vi "Polynomial Eigenvalues and Vectors (CDB).vi"(10 "output option":i32(ring)=1 items=["eigenvalues", "eigenvalues & vectors"], 11 "Input Matrices":cdb[][][](array[numeric])) -> (0 "error":i32, 2 "Eigenvectors":T1, 3 "Eigenvalues":cdb[](array[numeric]))   [LabVIEW 2010, in "NI_AALPro.lvlib"]
doc: "Solves the polynomial eigenvalue problem. Wire data to the <B>Input Matrices</B> input to determine the polymorphic instance to use or manually select the instance."
uses:
  NI_AALPro.lvlib
  ComplexMatrix.ctl
  NI_Matrix.lvlib
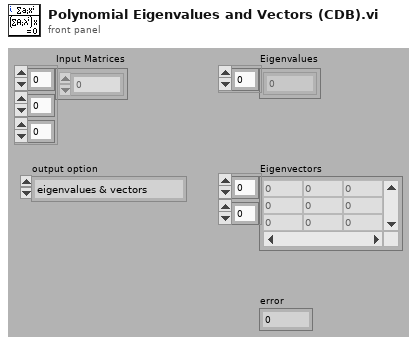
[diagram p1: front panel]
types:
  T1 = typedef "NI_Matrix.lvlib/ComplexMatrix.ctl" = cdb[][]
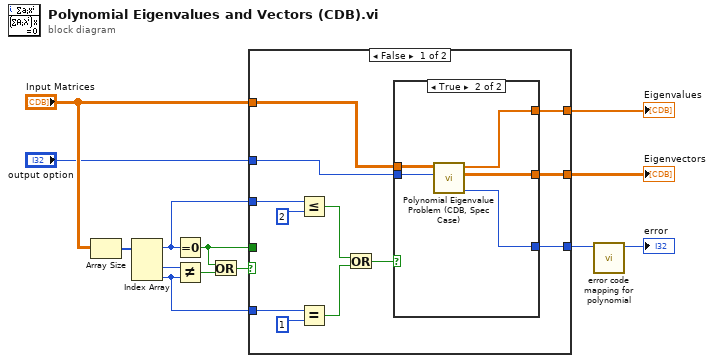
[diagram p0: block diagram]
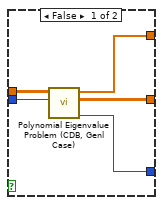
[diagram p2: hidden frame]
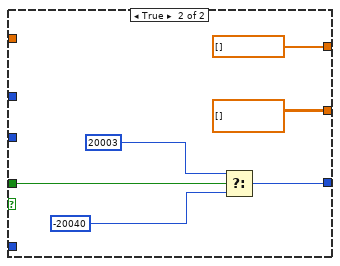
[diagram p3: hidden frame]
diagram:
  n1 = Array Size(array="Input Matrices") -> (size(s)=w13:i32[])
  n2 = Index Array(array=w13) -> (element #1=w7:i32, element #2=w12:i32, element #3=w8:i32)  [unwired: 3 in]
  n3 = Equal To 0?(x=w7) -> (x = 0?=w9:bool)
  n4 = Not Equal?(x=w12, y=w8) -> (x != y?=w11:bool)
  n5 = Or(x=w9, y=w11) -> (x .or. y?=w10:bool)
  n6 = case shown="False" w10 {
    tunnel: w9 -> [_ w41]
    tunnel: [w15 w38] -> w2
    tunnel: [w17 cdb[] [] ("Eigenvectors")] -> w4
    tunnel: [w16 cdb[][] [] ("Eigenvectors")] -> w5
    tunnel: "Input Matrices" -> [w23 _]
    tunnel: w8 -> [w25 _]
    tunnel: w7 -> [w22 _]
    tunnel: "output option" -> [w14 _]
    frame False {
      n7 = Less Or Equal?(x=w22, y=2) -> (x <= y?=w20:bool)
      n8 = Equal?(x=w25, y=1) -> (x = y?=w19:bool)
      n9 = Or(x=w20, y=w19) -> (x .or. y?=w18:bool)
      n10 = case shown="True" w18 {
        tunnel: w23 -> [w30 w35]
        tunnel: [w29 w34] -> w17
        tunnel: [w28 w33] -> w16
        tunnel: [w27 w32] -> w15
        tunnel: w14 -> [w26 w31]
        frame False {
          n11 = call "Polynomial Eigenvalue Problem (CDB, Genl Case).vi"("output option"=w26, "Input Matrices"=w30) -> ("error"=w27:i32, "Eigenvectors"=w28:T1, "Eigenvalues"=w29:cdb[])  [unwired: 7 in]
        }
        frame True {
          n12 = call "Polynomial Eigenvalue Problem (CDB, Spec Case).vi"("output option"=w31, "Input Matrices"=w35) -> ("error"=w32:i32, "Eigenvectors"=w33:T1, "Eigenvalues"=w34:cdb[])  [unwired: 7 in]
        }
      }
    }
    frame True {
      n13 = Select(t=20003 ("empty array"), s=w41, f=-20040 ("not a square matrix")) -> (s? t:f=w38:i32)
    }
  }
  "Eigenvectors" <- w5
  "Eigenvalues" <- w4
  n14 = call "error code mapping for polynomial.vi"("error in"=w2) -> ("error out"=→"error":i32)  [unwired: 10 in]
